vi "Read Count Measurement (Serial Bus - Flexray).vi"(8 "error in (no error)":errorcluster, 10 "Serial Bus Name (1: Serial Bus 1)":i32(ring)=1 items=["Serial Bus 1"=1, "Serial Bus 2"=2], 11 "VISA resource name":refnum<visa-resource-name>) -> (0 "error out":errorcluster, 1 "Sync Frame Count":dbl, 2 "Null Frame Count":dbl, 3 "VISA resource name out":refnum<visa-resource-name>, 5 "Total Frame Count":dbl)   [LabVIEW 2017, in "Agilent 2000 3000 X-Series.lvlib"]
doc: "Returns the measurement of serial bus - FlexRay.\n\nNote:\nThis VI is not supported by EDUX1052A, EDUX1052G, DSOX1202A, DSOX1202G, DSOX1204A, DSOX1204G models"
uses:
  Agilent 2000 3000 X-Series.lvlib
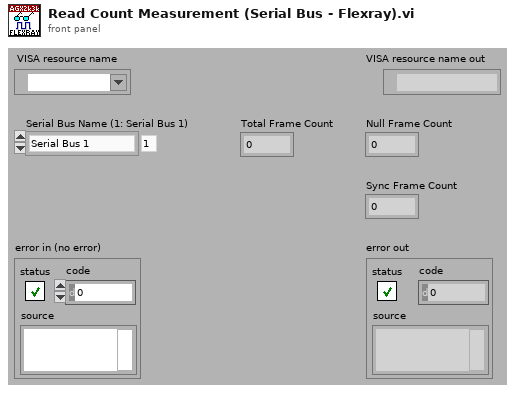
[diagram p1: front panel]
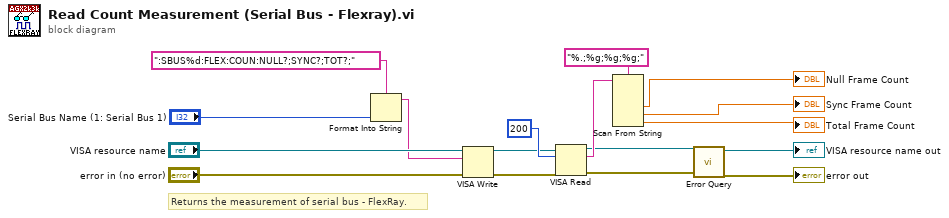
[diagram p0: block diagram]
diagram:
  # "Returns the measurement of serial bus - FlexRay."
  n1 = Format Into String(format string=":SBUS%d:FLEX:COUN:NULL?;SYNC?;TOT?;", "Serial Bus Name (1: Serial Bus 1)") -> (resulting string=w1:string)  [unwired: 2 in, 1 out]
  n2 = VISA Write(VISA resource name="VISA resource name", write buffer=w1, error in (no error)="error in (no error)") -> (VISA resource name out=w9:refnum<visa-resource-name>, error out=w8:errorcluster)  [unwired: 1 out]
  n3 = VISA Read(VISA resource name=w9, byte count=u32 200, error in (no error)=w8) -> (VISA resource name out=w6:refnum<visa-resource-name>, read buffer=w10:string, error out=w7:errorcluster)  [unwired: 1 out]
  n4 = Scan From String(format string="%.;%g;%g;%g;", input string=w10) -> (output 1=→"Null Frame Count":dbl, output 2=→"Sync Frame Count":dbl, output 3=→"Total Frame Count":dbl)  [unwired: 2 in, 6 out]
  n5 = call "Error Query.vi"("error in (no error)"=w7, "VISA resource name"=w6) -> ("error out"=→"error out":errorcluster, "VISA resource name out"=→"VISA resource name out":refnum<visa-resource-name>)  [unwired: 8 out]
